vi "New.vi"(8 "error in (no error)":errorcluster, 10 "Text":string, 11 "Path (\"\")":path) -> (0 "error out":errorcluster, 3 "Config":T1)   [LabVIEW 2022 SP3, in "LabVIEW-Config.lvlib"]
uses:
  LabVIEW-Config.lvlib
  Config.ctl
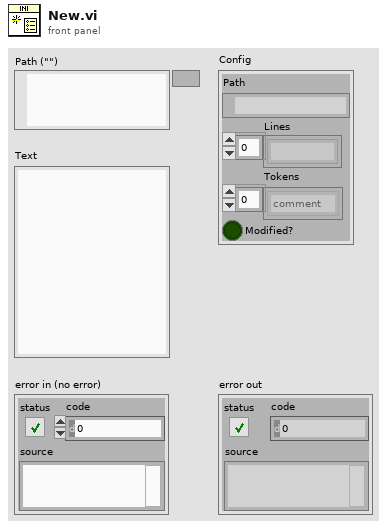
[diagram p1: front panel]
types:
  T1 = typedef "LabVIEW-Config.lvlib/Config.ctl" = cluster{"Path":path, "Lines":string[], "Tokens":enum8{"comment", "section", "key"}[], "Modified?":bool}
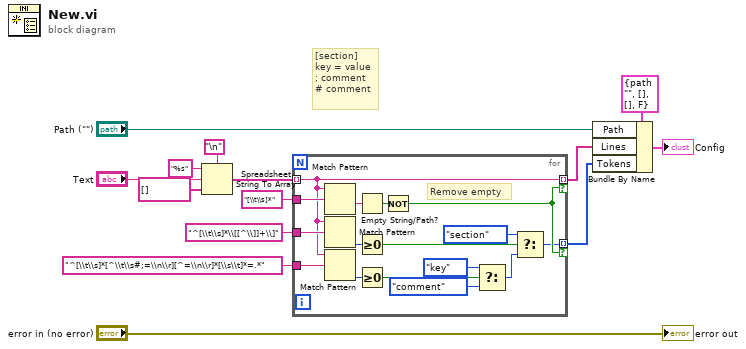
[diagram p0: block diagram]
diagram:
  # "[section]\nkey = value\n; comment\n# comment"
  n1 = Spreadsheet String To Array(delimiter (Tab)="\n" ("Line Feed Constant"), format string="%s", spreadsheet string="Text", array type (2D Dbl)=string[] []) -> (array=w1:string[])
  n2 = for {
    tunnel: w1 -> [w25] mode=indexing
    tunnel: "^[\\t\\s]*\\[[^\\]]+\\]" ("regular expression") -> [w30]
    tunnel: [w15] -> w9 mode=indexing if=w22
    tunnel: "^[\\t\\s]*[^\\t\\s#;=\\n\\r][^=\\n\\r]*[\\s\\t]*=.*" ("regular expression") -> [w24]
    tunnel: "[\\t\\s]*" ("regular expression") -> [w28]
    tunnel: [w25] -> w5 mode=indexing if=w22
    # "Remove empty"
    n3 = Match Pattern(string=w25, regular expression=w28) -> (after substring=w29:string)  [unwired: 1 in, 3 out]
    n4 = Match Pattern(string=w25, regular expression=w30) -> (offset past match=w27:i32)  [unwired: 1 in, 3 out]
    n5 = Match Pattern(string=w25, regular expression=w24) -> (offset past match=w26:i32)  [unwired: 1 in, 3 out]
    n6 = Empty String/Path?(string/path=w29) -> (empty?=w23:bool)
    n7 = Greater Or Equal To 0?(x=w27) -> (x >= 0?=w21:bool)
    n8 = Greater Or Equal To 0?(x=w26) -> (x >= 0?=w17:bool)
    n9 = Not(x=w23) -> (.not. x?=w22:bool)
    n10 = Select(t=enum8{"comment", "section", "key"}."key" ("Token"), s=w17, f=enum8{"comment", "section", "key"}."comment" ("Token")) -> (s? t:f=w18:enum8{"comment", "section", "key"})
    n11 = Select(t=enum8{"comment", "section", "key"}."section" ("Token"), s=w21, f=w18) -> (s? t:f=w15:enum8{"comment", "section", "key"})
  }
  n12 = Bundle By Name(cluster=T1 {"Path"=path "", "Lines"=[], "Tokens"=[], "Modified?"=FALSE} ("Refnum"), "Path"="Path (\"\")", "Lines"=w5, "Tokens"=w9) -> (→"Config":T1)
  "error out" <- "error in (no error)"
